vi "EnFlo_Seeder_Control.vi"(0 "Current Time (s)":dbl) -> ()   [LabVIEW 2012]
panel:
  in  "Performing hand clean":bool
  out "Run Transducer":bool
  out "Sugar Pump":bool
  out "Low Flow":bool
  out "High Flow":bool
  out "Time Since Last Flush (min)":dbl
  out "Running Flush time":dbl
  out "Transducer setting":dbl
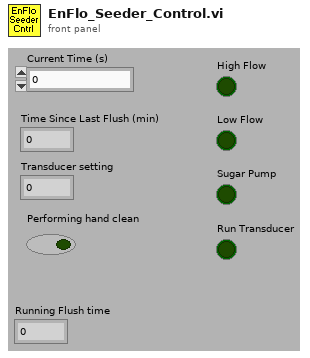
[diagram p1: front panel]
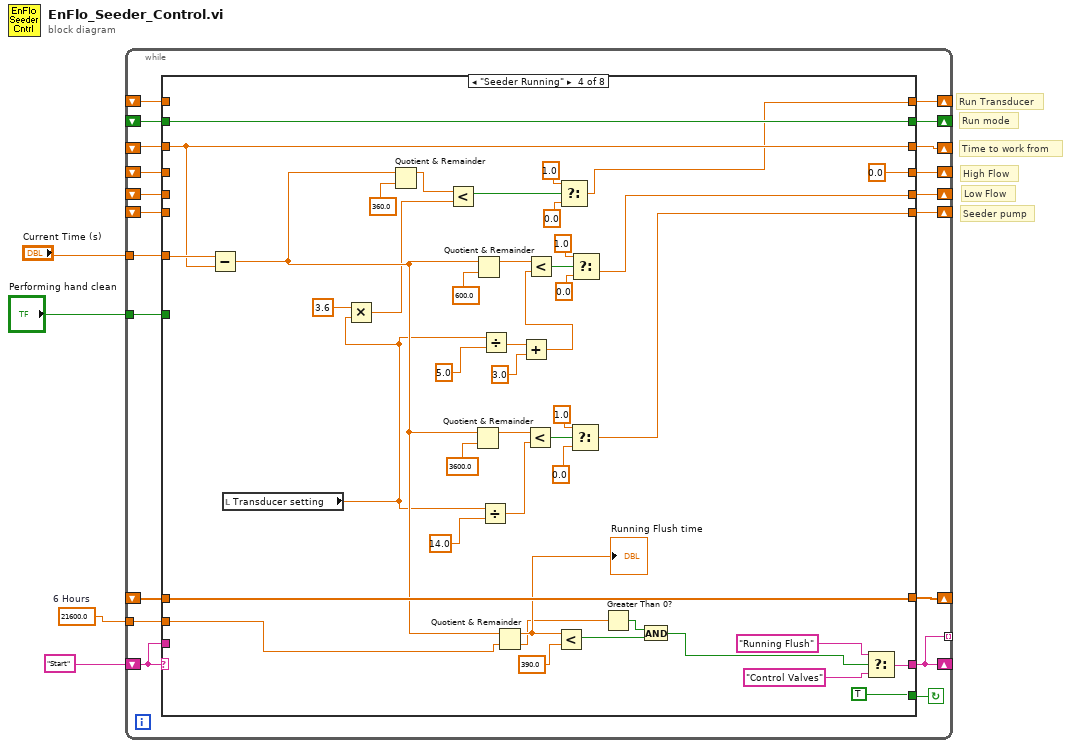
[diagram p0: block diagram]
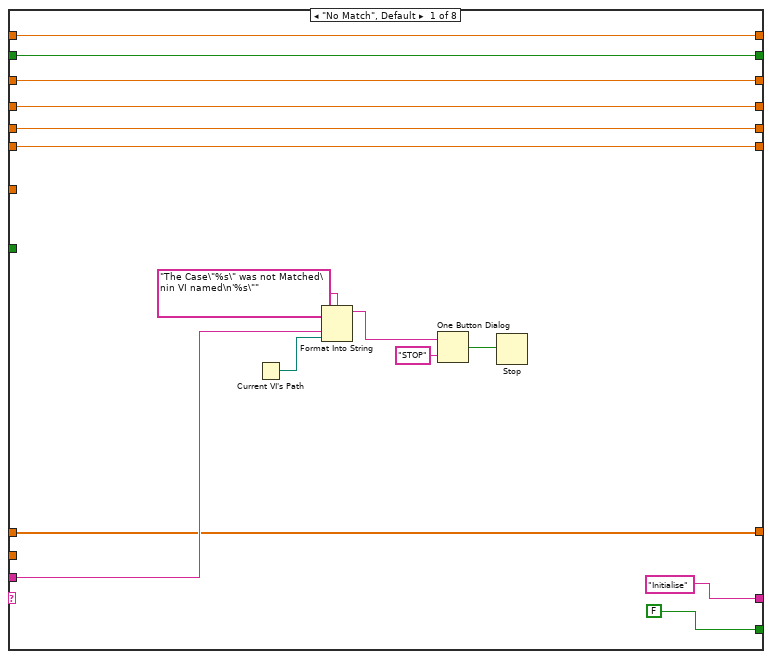
[diagram p2: hidden frame]
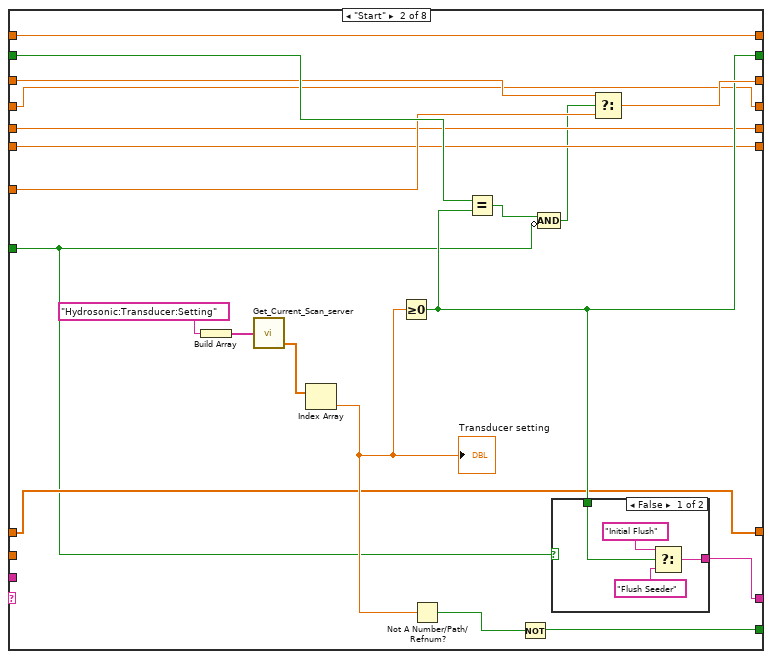
[diagram p3: hidden frame]
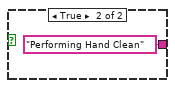
[diagram p4: hidden frame]
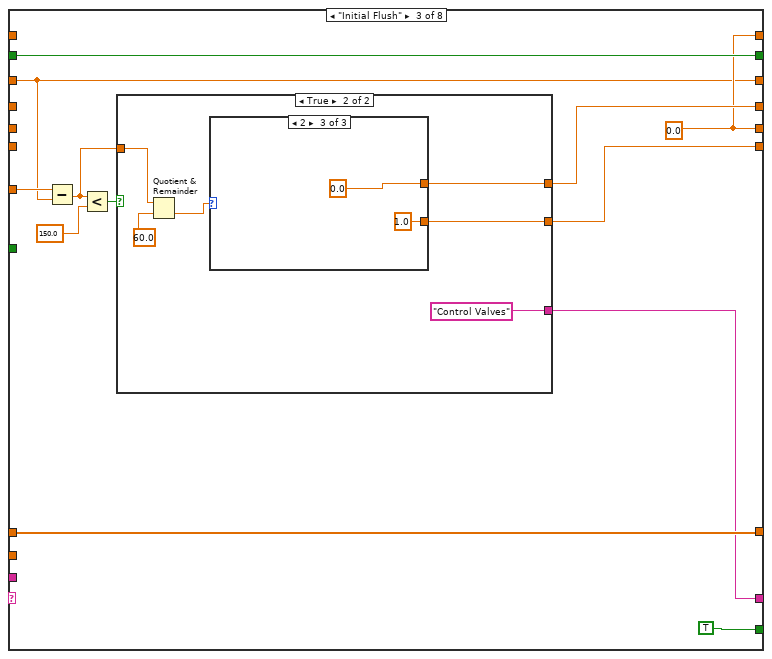
[diagram p5: hidden frame]
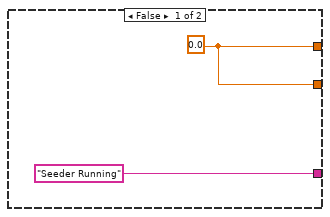
[diagram p6: hidden frame]
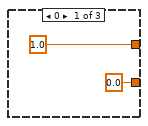
[diagram p7: hidden frame]
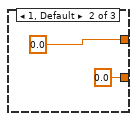
[diagram p8: hidden frame]
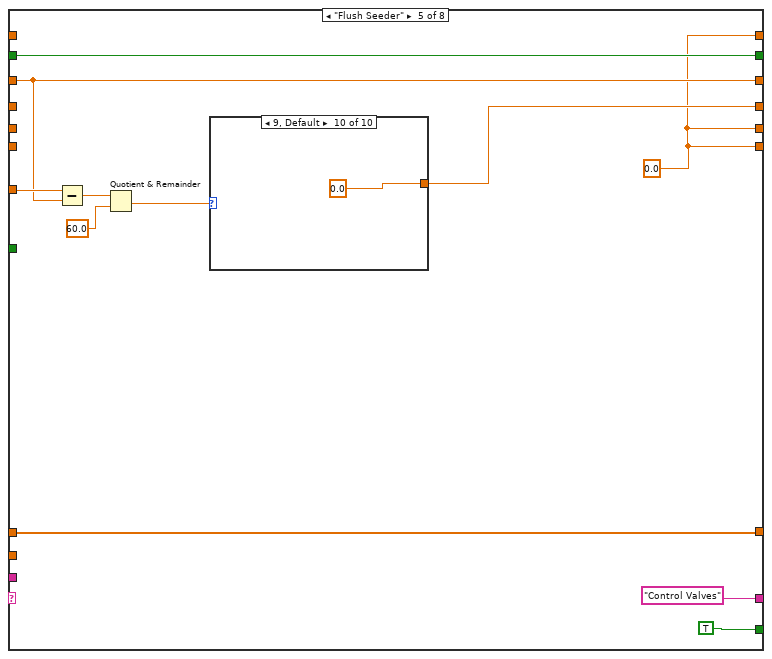
[diagram p9: hidden frame]
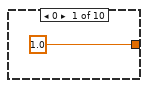
[diagram p10: hidden frame]
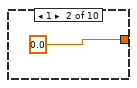
[diagram p11: hidden frame]
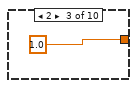
[diagram p12: hidden frame]
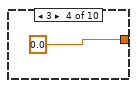
[diagram p13: hidden frame]
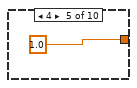
[diagram p14: hidden frame]
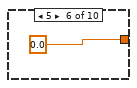
[diagram p15: hidden frame]
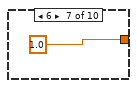
[diagram p16: hidden frame]
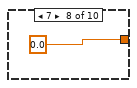
[diagram p17: hidden frame]
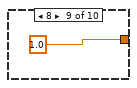
[diagram p18: hidden frame]
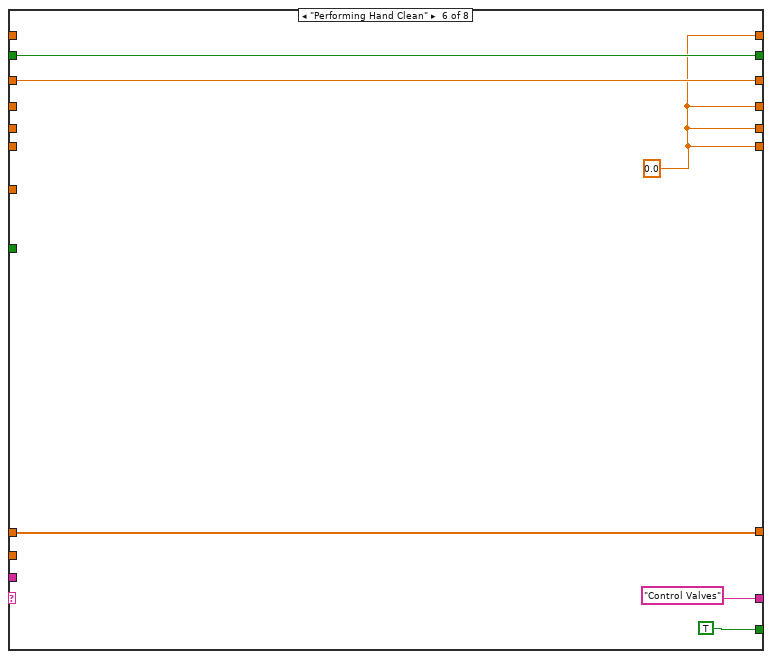
[diagram p19: hidden frame]
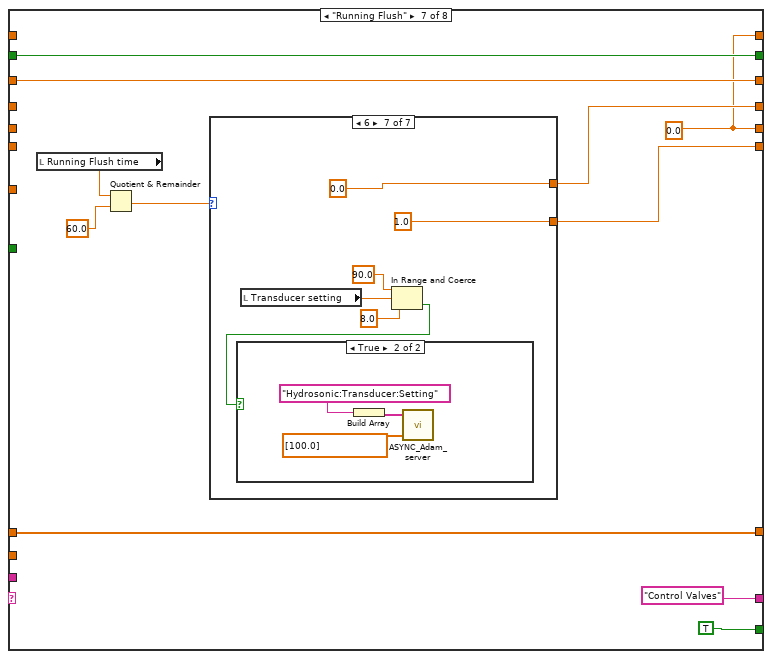
[diagram p20: hidden frame]
diagram:
  w2 = 21600.0  # 6 Hours
  # "Run Transducer"
  # "Seeder pump"
  # "Low Flow"
  # "High Flow"
  # "Run mode"
  # "Time to work from"
  n1 = while {
    shift-left: "Start" -> [w23]
    shift-right: [w7] -> _
    shift-right: [w22] -> _
    shift-left: _ -> [w19]
    shift-right: [w21] -> _
    shift-left: _ -> [w20]
    tunnel: "Current Time (s)" -> [w18]
    shift-right: [w16] -> _
    shift-left: _ -> [w17]
    shift-right: [w15] -> _
    shift-left: _ -> [w14]
    shift-right: [w12] -> _
    shift-left: _ -> [w13]
    shift-right: [w10] -> _
    shift-left: _ -> [w11]
    shift-right: [w9] -> _
    shift-left: _ -> [w8]
    tunnel: [w7] -> _ mode=indexing
    tunnel: w2 -> [w6]
    tunnel: "Performing hand clean" -> [w5]
    stop <- w24 continue-if-true
    n2 = case shown="\"Seeder Running\"" w23 {
      tunnel: [FALSE w55 TRUE TRUE TRUE TRUE TRUE FALSE] -> w24
      tunnel: ["Initialise" w48 w65 w108 "Control Valves" "Control Valves" "Control Valves" "End"] -> w7
      tunnel: w23 -> [w34 _ _ _ _ _ _ _]
      tunnel: [w29 w52 w69 w132 w141 w158 w169 w210] -> w22
      tunnel: [w31 w49 w75 w134 w143 w159 w170 w220] -> w21
      tunnel: w20 -> [w31 w53 w75 w134 w143 w159 w170 w220]
      tunnel: w19 -> [w29 w51 w69 w132 w141 w158 w169 w210]
      tunnel: w18 -> [_ w50 w70 w133 w142 _ _ w211]
      tunnel: w17 -> [w30 w47 _ _ _ _ _ w207]
      tunnel: [w30 w47 w74 0.0 w137 w156 w166 w207] -> w16
      tunnel: w14 -> [w28 w45 _ _ _ _ _ w205]
      tunnel: [w28 w45 w71 w120 w135 w156 w162 w205] -> w15
      tunnel: w13 -> [w27 w44 _ _ _ _ _ w203]
      tunnel: [w27 w44 w72 w112 w135 w156 w163 w203] -> w12
      tunnel: w11 -> [w26 w46 w73 w130 w136 w157 w165 w199]
      tunnel: [w26 w46 w73 w130 w136 w157 w165 w219] -> w10
      tunnel: w8 -> [w25 w43 _ _ _ _ _ w201]
      tunnel: [w25 w43 w71 w97 w135 w156 w162 w201] -> w9
      tunnel: w6 -> [_ _ _ w91 _ _ _ w195]
      tunnel: w5 -> [_ w40 _ _ _ _ _ _]
      frame "No Match", Default {
        n3 = Current VI's Path() -> (path=w33:path)
        n4 = Format Into String(format string="The Case\"%s\" was not Matched\nin VI named\n'%s\"" ("Format String"), w34, w33) -> (resulting string=w37:string)  [unwired: 2 in, 1 out]
        n5 = One Button Dialog(message=w37, button name ("OK")="STOP") -> (true=w35:bool)
        n6 = Stop(stop? (T)=w35) -> ()
      }
      frame "Start" {
        n7 = Build Array("Hydrosonic:Transducer:Setting") -> (w58:string[])
        n8 = call "Get_Current_Scan_server.vi"("Desired Channels"=w58) -> ("Numerical Values"=w57:dbl[])  [unwired: 2 out]
        n9 = Index Array(array=w57) -> (element=w54:dbl)  [unwired: 1 in]
        "Transducer setting" <- w54
        n10 = Greater Or Equal To 0?(x=w54) -> (x >= 0?=w49:bool)
        n11 = Not A Number/Path/Refnum?(number/path/refnum=w54) -> (NaN/Path/Refnum?=w56:bool)
        n12 = Equal?(x=w53, y=w49) -> (x = y?=w42:bool)
        n13 = Not(x=w56) -> (.not. x?=w55:bool)
        n14 = Compound Arithmetic op=AND(w42, invert w40) -> (w41:bool)
        n15 = case shown="False" w40 {
          tunnel: w49 -> [w63 _]
          tunnel: [w62 "Performing Hand Clean"] -> w48
          frame False {
            n16 = Select(t="Initial Flush", s=w63, f="Flush Seeder") -> (s? t:f=w62:string)
          }
          frame True {
          }
        }
        n17 = Select(t=w51, s=w41, f=w50) -> (s? t:f=w52:dbl)
      }
      frame "Initial Flush" {
        w71 = 0.0
        n18 = Subtract(x=w70, y=w69) -> (x-y=w66:dbl)
        n19 = Less?(x=w66, y=150.0) -> (x < y?=w67:bool)
        n20 = case shown="True" w67 {
          tunnel: [w78 w84] -> w74
          tunnel: [w78 w83] -> w72
          tunnel: w66 -> [_ w81]
          tunnel: ["Seeder Running" "Control Valves"] -> w65
          frame False {
            w78 = 0.0
          }
          frame True {
            n21 = Quotient & Remainder(x=w81, y=60.0) -> (floor(x/y)=w80:dbl)  [unwired: 1 out]
            n22 = case shown="2" w80 {
              tunnel: [1.0 0.0 0.0] -> w84
              tunnel: [0.0 0.0 1.0] -> w83
              frame 0 {
              }
              frame 1, Default {
              }
              frame 2 {
              }
            }
          }
        }
      }
      frame "Seeder Running" {
        n23 = Subtract(x=w133, y=w132) -> (x-y=w105:dbl)
        n24 = local read "Transducer setting"() -> (w104:dbl)
        n25 = Multiply(x=3.6, y=w104) -> (x*y=w101:dbl)
        n26 = Quotient & Remainder(x=w105, y=360.0) -> (x-y*floor(x/y)=w102:dbl)  [unwired: 1 out]
        n27 = Less?(x=w102, y=w101) -> (x < y?=w98:bool)
        n28 = Quotient & Remainder(x=w105, y=3600.0) -> (x-y*floor(x/y)=w115:dbl)  [unwired: 1 out]
        n29 = Quotient & Remainder(x=w105, y=600.0) -> (x-y*floor(x/y)=w129:dbl)  [unwired: 1 out]
        n30 = Divide(x=w104, y=14.0) -> (x/y=w113:dbl)
        n31 = Divide(x=w104, y=5.0) -> (x/y=w125:dbl)
        n32 = Quotient & Remainder(x=w105, y=w91) -> (x-y*floor(x/y)=w107:dbl, floor(x/y)=w95:dbl)
        "Running Flush time" <- w107
        n33 = Add(x=w125, y=3.0) -> (x+y=w123:dbl)
        n34 = Less?(x=w115, y=w113) -> (x < y?=w116:bool)
        n35 = Less?(x=w129, y=w123) -> (x < y?=w128:bool)
        n36 = Less?(x=w107, y=390.0) -> (x < y?=w93:bool)
        n37 = Select(t=1.0, s=w98, f=0.0) -> (s? t:f=w97:dbl)
        n38 = Select(t=1.0, s=w116, f=0.0) -> (s? t:f=w112:dbl)
        n39 = Select(t=1.0, s=w128, f=0.0) -> (s? t:f=w120:dbl)
        n40 = Greater Than 0?(x=w95) -> (x > 0?=w94:bool)
        n41 = And(x=w94, y=w93) -> (x .and. y?=w92:bool)
        n42 = Select(t="Running Flush", s=w92, f="Control Valves") -> (s? t:f=w108:string)
      }
      frame "Flush Seeder" {
        w135 = 0.0
        n43 = Subtract(x=w142, y=w141) -> (x-y=w140:dbl)
        n44 = Quotient & Remainder(x=w140, y=60.0) -> (floor(x/y)=w138:dbl)  [unwired: 1 out]
        n45 = case shown="9, Default" w138 {
          tunnel: [1.0 0.0 1.0 0.0 1.0 0.0 1.0 0.0 1.0 0.0] -> w137
          frame 0 {
          }
          frame 1 {
          }
          frame 2 {
          }
          frame 3 {
          }
          frame 4 {
          }
          frame 5 {
          }
          frame 6 {
          }
          frame 7 {
          }
          frame 8 {
          }
          frame 9, Default {
          }
        }
      }
      frame "Performing Hand Clean" {
        w156 = 0.0
      }
      frame "Running Flush" {
        w162 = 0.0
        n46 = local read "Running Flush time"() -> (w164:dbl)
        n47 = Quotient & Remainder(x=w164, y=60.0) -> (floor(x/y)=w167:dbl)  [unwired: 1 out]
        n48 = case shown="6" w167 {
          tunnel: [1.0 0.0 1.0 0.0 1.0 0.0 0.0] -> w166
          tunnel: [0.0 0.0 0.0 0.0 0.0 0.0 1.0] -> w163
          frame 0 {
          }
          frame 1 {
          }
          frame 2 {
          }
          frame 3 {
          }
          frame 4 {
          }
          frame 5, Default {
          }
          frame 6 {
            n49 = local read "Transducer setting"() -> (w188:dbl)
            n50 = In Range and Coerce(upper limit=90.0, x=w188, lower limit=8.0) -> (In Range?=w185:bool)  [unwired: 1 out]
            n51 = case shown="True" w185 {
              frame False {
              }
              frame True {
                n52 = Build Array("Hydrosonic:Transducer:Setting") -> (w192:string[])
                n53 = call "ASYNC_Adam_server.vi"("Values"=dbl[] [100.0], "Channel Names"=w192) -> ()  [unwired: 1 in, 3 out]
              }
            }
          }
        }
      }
      frame "Control Valves" {
        n54 = Subtract(x=w211, y=w210) -> (x-y=w196:dbl)
        n55 = Quotient & Remainder(x=w196, y=w195) -> (x-y*floor(x/y)=w194:dbl)  [unwired: 1 out]
        n56 = Divide(x=w194, y=60.0) -> (x/y=→"Time Since Last Flush (min)":dbl)
        n57 = Build Array(w201, w207, w205, w203) -> (w219:dbl[])
        n58 = Array Size(array=w199) -> (size(s)=w198:i32)
        n59 = Equal To 0?(x=w198) -> (x = 0?=w197:bool)
        n60 = case shown="True" w197 {
          tunnel: w219 -> [w225 w230]
          tunnel: string[] ["Hydrosonic:Seeder:Enable", "EnFlo_Tunnel:Seeder:High_Flow", "EnFlo_Tunnel:Seeder:Low_Flow", "EnFlo_Tunnel:Seeder_Pump:Enable"] ("Desired Ch Names") -> [w224 w231]
          tunnel: [w223 w231] -> w215
          tunnel: [w222 w230] -> w214
          tunnel: w199 -> [w221 _]
          frame False {
            n61 = for {
              tunnel: w221 -> [w229] mode=indexing
              tunnel: w225 -> [w228] mode=indexing
              tunnel: [w228] -> w222 mode=indexing if=w226
              tunnel: w224 -> [w227] mode=indexing
              tunnel: [w227] -> w223 mode=indexing if=w226
              n62 = Not Equal?(x=w228, y=w229) -> (x != y?=w226:bool)
            }
          }
          frame True {
          }
        }
        n63 = Array Size(array=w214) -> (size(s)=w218:i32)
        n64 = Greater Than 0?(x=w218) -> (x > 0?=w217:bool)
        n65 = case shown="True" w217 {
          tunnel: w214 -> [_ w233]
          tunnel: w215 -> [_ w232]
          frame False {
          }
          frame True {
            n66 = call "ASYNC_Adam_server.vi"("Values"=w233, "Channel Names"=w232) -> ()  [unwired: 1 in, 3 out]
          }
        }
        n67 = Greater Than 0?(x=w207) -> (x > 0?=→"High Flow":bool)
        n68 = Greater Than 0?(x=w205) -> (x > 0?=→"Low Flow":bool)
        n69 = Greater Than 0?(x=w201) -> (x > 0?=→"Run Transducer":bool)
        n70 = Greater Than 0?(x=w203) -> (x > 0?=→"Sugar Pump":bool)
      }
    }
  }
